vi "GetTime.vi"(2 "error in (no error)":errorcluster) -> (0 "error out":errorcluster, 1 "CurrentTime":timestamp)   [LabVIEW 2009]
doc: "Get Current TIme"
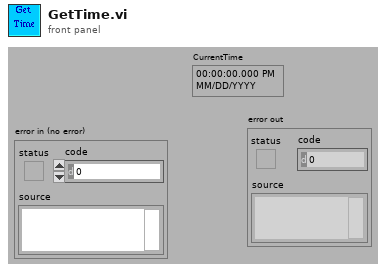
[diagram p1: front panel]
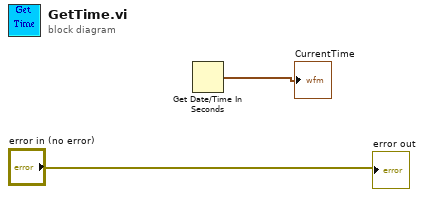
[diagram p0: block diagram]
diagram:
  n1 = Get Date/Time In Seconds() -> (seconds since 1Jan1904=→"CurrentTime":timestamp)
  "error out" <- "error in (no error)"
